vi "Assign Link Bounds.vi"(8 "error in (no error)":errorcluster, 11 "Link in":refnum<class "Link.lvclass">) -> (0 "error out":errorcluster, 3 "Link out":refnum<class "Link.lvclass">)   [LabVIEW 2017, in "LV Image Editor Framework.lvlib" / "Link.lvclass"]
uses:
  <vilib>/LIEF/Forms/Link/Link.lvclass
  C:/Github/LIEF/Forms/Shape/Shape.lvclass
  <vilib>/LIEF/Forms/Link/Link.lvclass/Link.ctl
  <vilib>/LIEF/Forms/Shape/Shape.lvclass
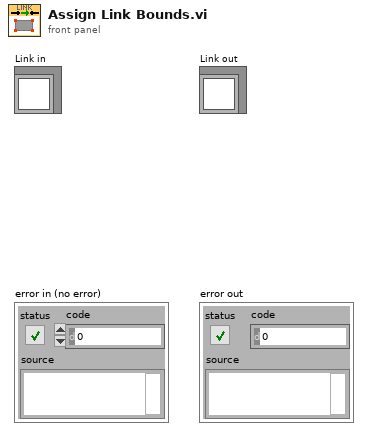
[diagram p1: front panel]
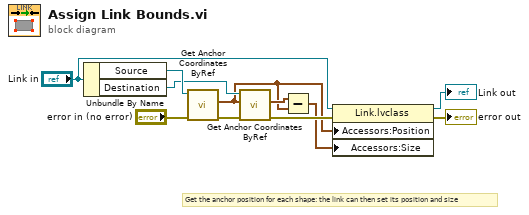
[diagram p0: block diagram]
diagram:
  # "Get the anchor position for each shape: the link can then set its position and size"
  n1 = Unbundle By Name("Link in") -> ("Source"=w3:refnum<data-value>, "Destination"=w2:refnum<data-value>)
  n2 = call <vilib>:"Get Anchor Coordinates ByRef.vi"("error in (no error)"="error in (no error)", "Shape Ref"=w3) -> ("error out"=w7:errorcluster, "Anchor Coords"=w1:cluster{"X":i32, "Y":i32})  [unwired: 7 in, 1 out]
  n3 = call <vilib>:"Get Anchor Coordinates ByRef.vi"("error in (no error)"=w7, "Raw Coords"=w1, "Shape Ref"=w2) -> ("error out"=w9:errorcluster, "Anchor Coords"=w5:cluster{"X":i32, "Y":i32})  [unwired: 6 in, 1 out]
  n4 = Subtract(x=w5, y=w1) -> (x-y=w6:cluster{"X":i32, "Y":i32})
  n5 = property class="Link.lvclass"(reference="Link in", error in=w9, "Accessors:Position"=w1, "Accessors:Size"=w6) -> (reference out=→"Link out":refnum<class "Link.lvclass">, error out=→"error out":errorcluster)
